vi "PXI-Set AI Config.vi"(0 "AI Channels":i32[](array[numeric]), 1 "Vmax":dbl=10.0, 2 "Vmin":dbl=-10.0, 5 "Sampling Rate (Hz)":dbl, 7 "Buffer Size":i32, 9 "Terminal configuration":i32(ring)=-1 items=["Default"=-1, "RSE"=10083, "Differential"=10106, "Pseudodifferential"=12529], 11 "error in (no error)":errorcluster, 12 "AI Transfer Mode":T1) -> (15 "error out":errorcluster)   [LabVIEW 2020]
uses:
  Type Defs/Channel Struct.ctl
  Type Defs/PXI-AI Transfer Mode.ctl
  DAQ Engine VIs/PXI Globals.vi
panel:
  in  "dummy chan struct":T2={"Channel name"="AI1", "Vmax"=10.0, "Vmin"=10.0, "Rate"=204800.0, "Terminal configuration"=-1, "Physical Channel"="", "Regenerate"=FALSE} {"Terminal configuration" items=["Default"=-1, "RSE"=10083, "Differential"=10106, "Pseudodifferential"=12529]}
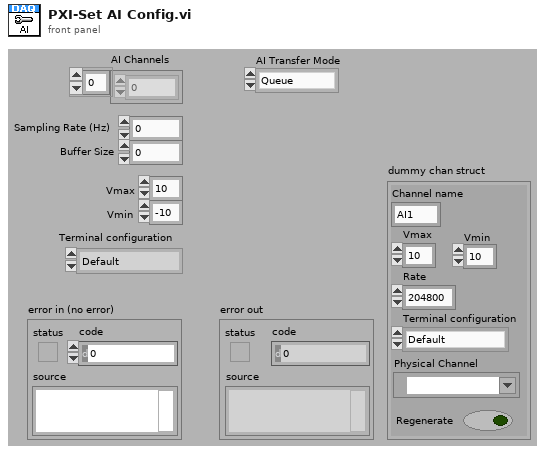
[diagram p1: front panel]
types:
  T1 = typedef "PXI-AI Transfer Mode.ctl" = enum16{"Queue", "Data Bank", "No Transfer"}
  T2 = typedef "Channel Struct.ctl" = cluster{"Channel name":string, "Vmax":dbl, "Vmin":dbl, "Rate":dbl, "Terminal configuration":i32, "Physical Channel":tag, "Regenerate":bool}
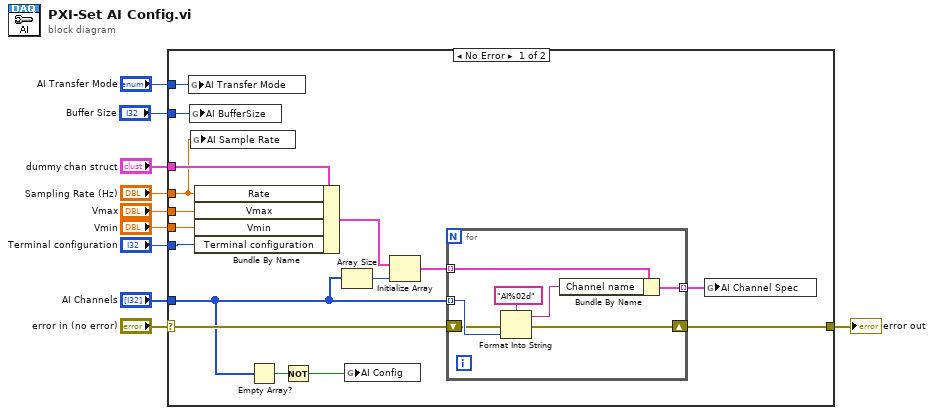
[diagram p0: block diagram]
diagram:
  n1 = case shown="No Error" "error in (no error)" {
    selector: "error in (no error)" -> [w18 w34]
    tunnel: "Terminal configuration" -> [w26 _]
    tunnel: "Vmin" -> [w25 _]
    tunnel: "Vmax" -> [w24 _]
    tunnel: "Sampling Rate (Hz)" -> [w15 _]
    tunnel: "dummy chan struct" -> [w23 _]
    tunnel: "AI Channels" -> [w12 _]
    tunnel: "Buffer Size" -> [w19 _]
    tunnel: [w17 w34] -> w2
    tunnel: "AI Transfer Mode" -> [w11 _]
    frame No Error {
      n2 = global write "PXI Globals.vi" "AI Transfer Mode"(w11) -> ()
      n3 = global write "PXI Globals.vi" "AI BufferSize"(w19) -> ()
      n4 = global write "PXI Globals.vi" "AI Sample Rate"(w15) -> ()
      n5 = Bundle By Name(cluster=w23, "Rate"=w15, "Vmax"=w24, "Vmin"=w25, "Terminal configuration"=w26) -> (w21:T2)
      n6 = Empty Array?(array=w12) -> (empty?=w14:bool)
      n7 = Not(x=w14) -> (.not. x?=w13:bool)
      n8 = Array Size(array=w12) -> (size(s)=w22:i32)
      n9 = global write "PXI Globals.vi" "AI Config"(w13) -> ()
      n10 = Initialize Array(w21, w22) -> (w20:T2[])
      n11 = for {
        tunnel: w12 -> [w32] mode=indexing
        tunnel: w20 -> [w31] mode=indexing
        tunnel: [w29] -> w16 mode=indexing
        shift-right: [w27] -> w17
        shift-left: w18 -> [w28]
        n12 = Format Into String(format string="AI%02d", error in=w28, w32) -> (resulting string=w30:string, error out=w27:errorcluster)  [unwired: 1 in]
        n13 = Bundle By Name(cluster=w31, "Channel name"=w30) -> (w29:T2)
      }
      n14 = global write "PXI Globals.vi" "AI Channel Spec"(w16) -> ()
    }
    frame Error {
    }
  }
  "error out" <- w2
